vi "Initialize.vi"(8 "Error In":errorcluster, 11 "Error Handling In":refnum<class "Error Handling.lvclass">) -> (0 "Error Out":errorcluster, 3 "Error Handling Out":refnum<class "Error Handling.lvclass">)   [LabVIEW 2019, in "Error Handling.lvclass"]
uses:
  Error Handling.lvclass
  Process/Process.lvclass
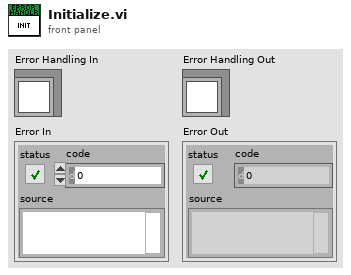
[diagram p1: front panel]
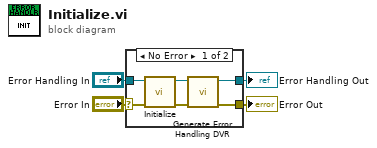
[diagram p0: block diagram]
diagram:
  n1 = case shown="No Error" "Error In" {
    selector: "Error In" -> [w10 w11]
    tunnel: [w5 w11] -> w4
    tunnel: [w6 w12] -> w3
    tunnel: "Error Handling In" -> [w9 w12]
    frame No Error {
      n2 = call-parent "Initialize.vi"("Error In"=w10, "Process In"=w9) -> ("Error Out"=w7:errorcluster, "Process Out"=w8:refnum<class "Error Handling.lvclass">)  [unwired: 8 in]
      n3 = call "Generate Error Handling DVR.vi"("Error In"=w7, "Error Handling In"=w8) -> ("Error Out"=w5:errorcluster, "Error Handling Out"=w6:refnum<class "Error Handling.lvclass">)  [unwired: 8 in]
    }
    frame Error {
    }
  }
  "Error Handling Out" <- w3
  "Error Out" <- w4
